vi "Cannon Speed Control.vi"(1 "Cannon Global Data In":T1) -> (0 "Cannon Global Data Out":T1)   [LabVIEW 2012]
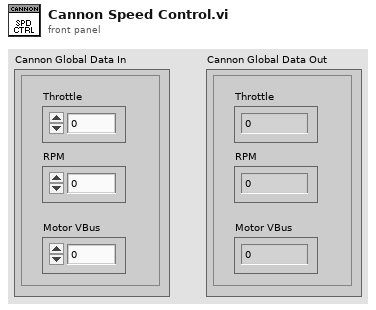
[diagram p1: front panel]
types:
  T1 = cluster{"Throttle":dbl, "RPM":dbl, "Motor VBus":dbl}
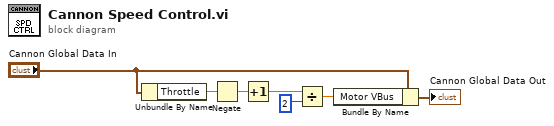
[diagram p0: block diagram]
diagram:
  n1 = Unbundle By Name("Cannon Global Data In") -> ("Throttle"=w2:dbl)
  n2 = Negate(x=w2) -> (-x=w3:dbl)
  n3 = Increment(x=w3) -> (x+1=w4:dbl)
  n4 = Divide(x=w4, y=2) -> (x/y=w1:dbl)
  n5 = Bundle By Name(cluster="Cannon Global Data In", "Motor VBus"=w1) -> (→"Cannon Global Data Out":T1)
